vi "Controller Apply BPM Configuration.vi"(8 "Inverse BPM Matrix Mapping":u32[][](array[numeric]), 9 "BPM Configuration Status Out":refnum<notifier>, 10 "BPM Configuration Status In":refnum<notifier>, 11 "Acquisition Network In":T1) -> (2 "Changed?":bool, 3 "Acquisition Network Out":T1)   [LabVIEW 2011, in "Controller VIs.lvlib"]
uses:
  Controller VIs.lvlib
  Types Definitions/Type Acquisition Network Configuration.ctl
  Type Definitions.lvlib
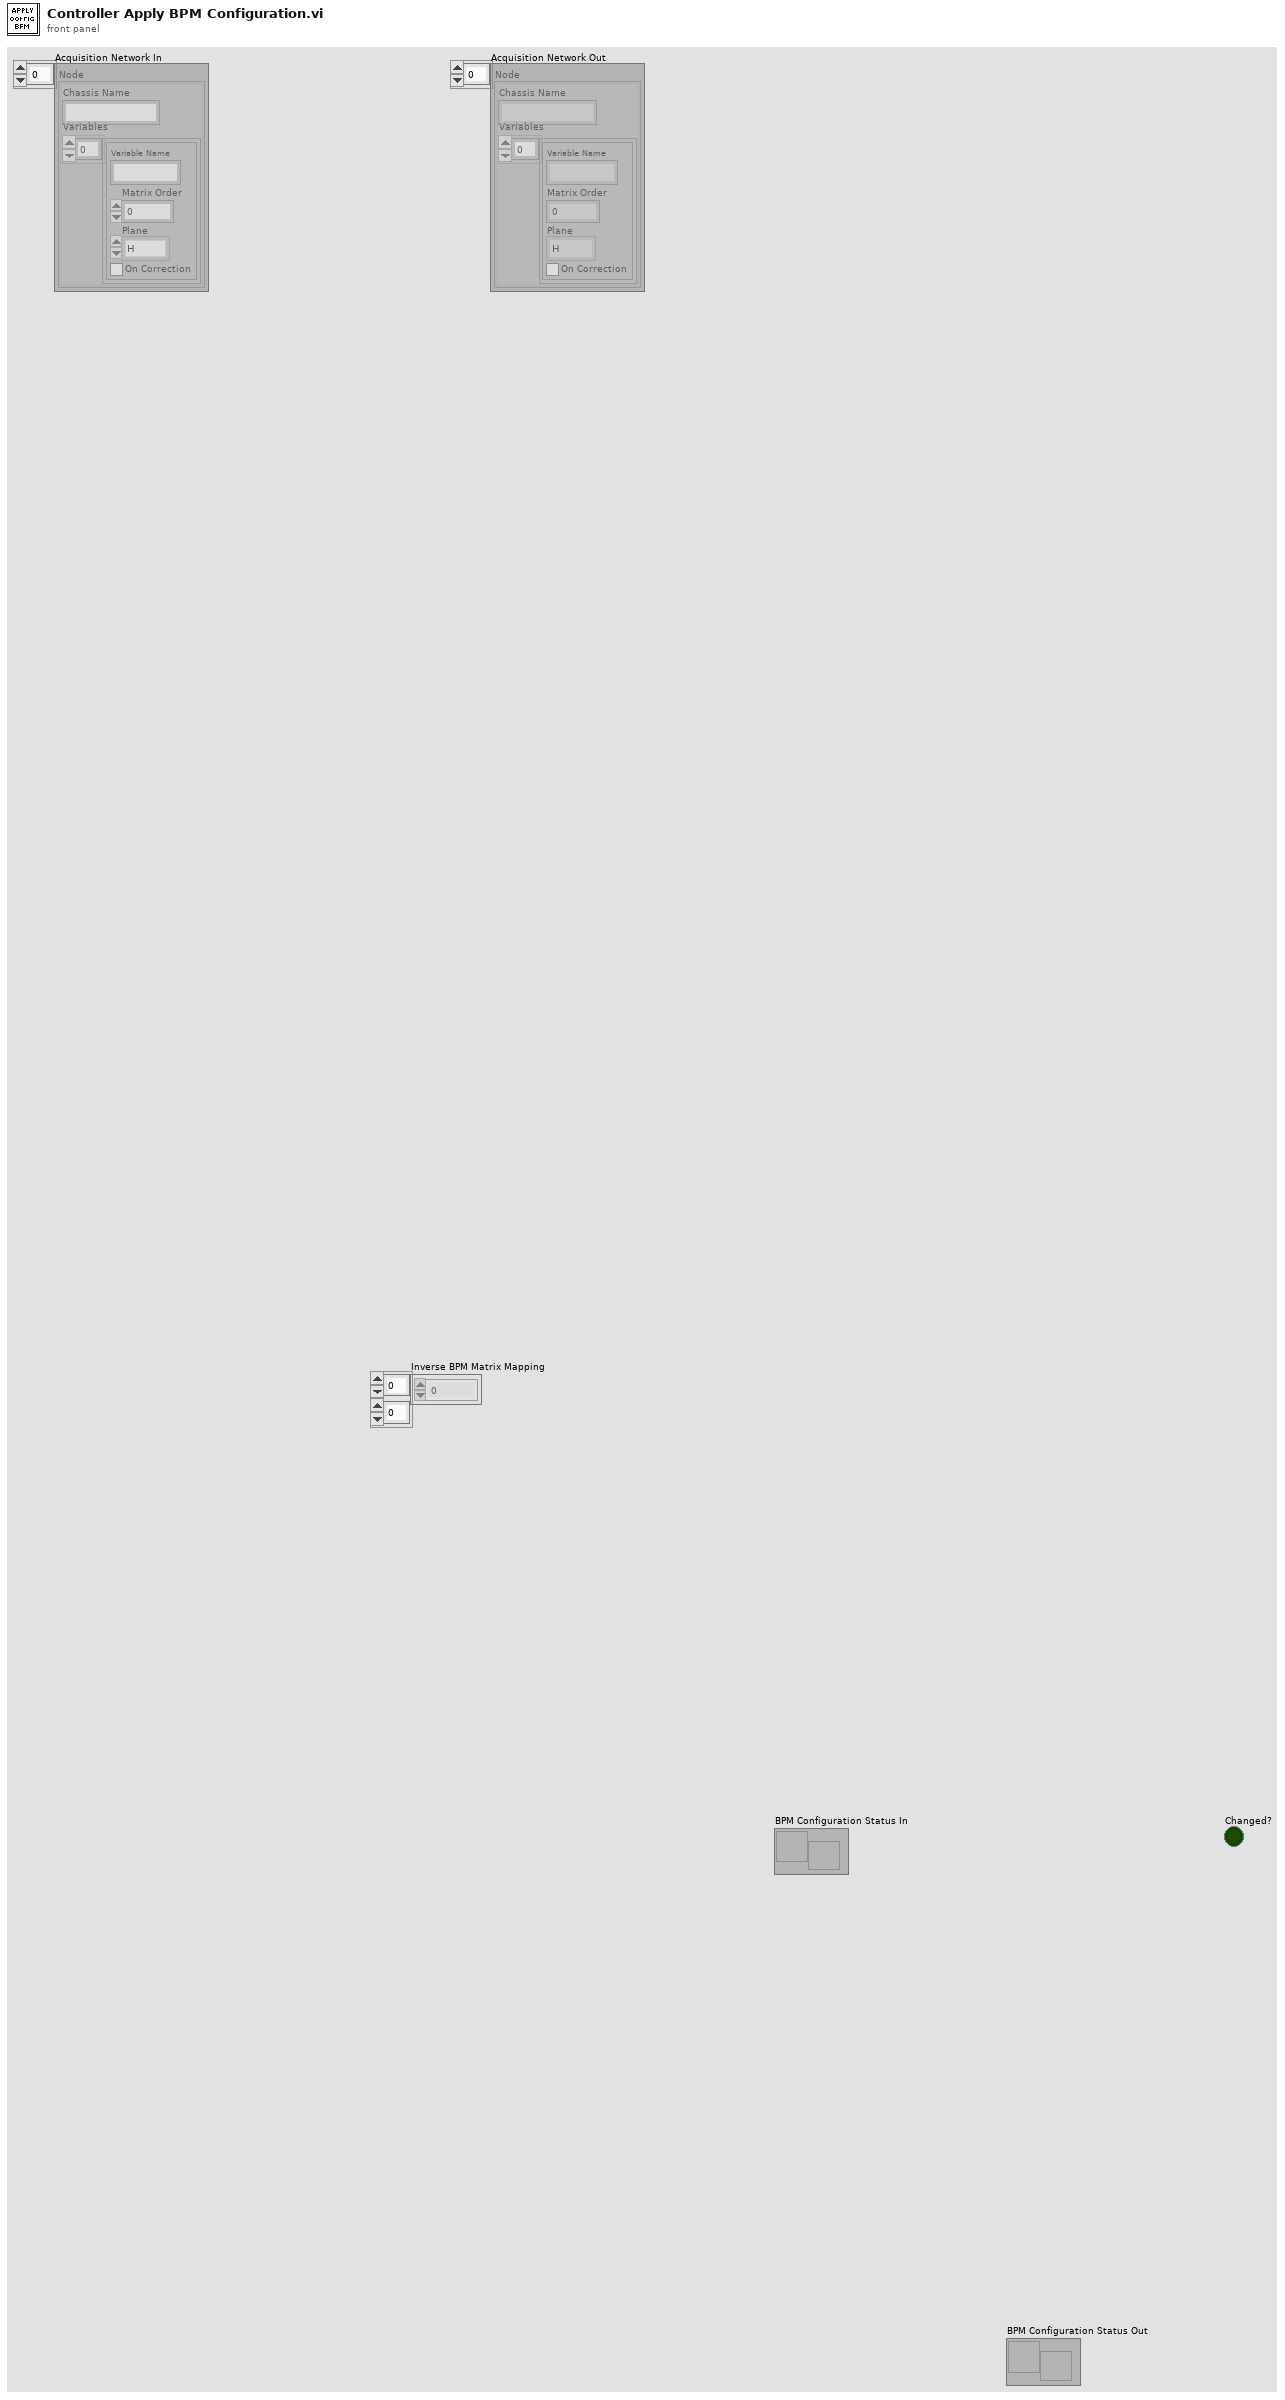
[diagram p1: front panel]
types:
  T1 = typedef "Type Definitions.lvlib/Type Acquisition Network Configuration.ctl" = cluster{"Chassis Name":string, "Variables":cluster{"Variable Name":string, "Matrix Order":u32, "Plane":enum8{"H", "V"}, "On Correction":bool}[]}[]
  T2 = cluster{"Chassis Name":string, "Variables":cluster{"Variable Name":string, "Matrix Order":u32, "Plane":enum8{"H", "V"}, "On Correction":bool}[]}
  T3 = cluster{"Variable Name":string, "Matrix Order":u32, "Plane":enum8{"H", "V"}, "On Correction":bool}[]
  T4 = cluster{"Variable Name":string, "Matrix Order":u32, "Plane":enum8{"H", "V"}, "On Correction":bool}
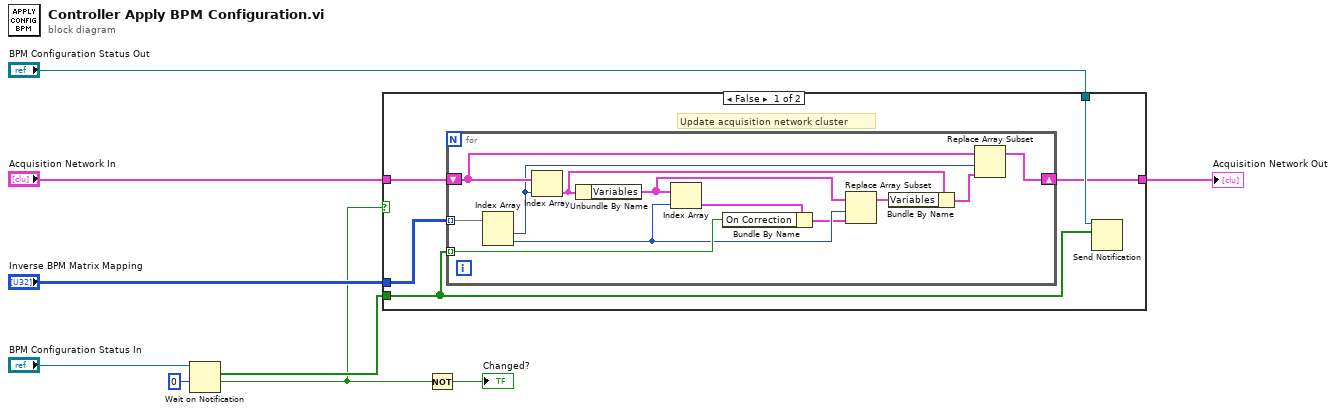
[diagram p0: block diagram]
diagram:
  n1 = Wait on Notification(notifier="BPM Configuration Status In", timeout in ms (-1)=0) -> (notification=w5:bool[], timed out?=w1:bool)  [unwired: 2 in, 2 out]
  n2 = case shown="False" w1 {
    tunnel: "Acquisition Network In" -> [w13 w27]
    tunnel: [w12 w27] -> w3
    tunnel: "BPM Configuration Status Out" -> [w14 _]
    tunnel: w5 -> [w10 _]
    tunnel: "Inverse BPM Matrix Mapping" -> [w11 _]
    frame False {
      # "Update acquisition network cluster"
      n3 = for {
        tunnel: w11 -> [w26] mode=indexing
        tunnel: w10 -> [w24] mode=indexing
        shift-right: [w15] -> w12
        shift-left: w13 -> [w23]
        n4 = Index Array(array=w26) -> (element #1=w22:u32, element #2=w20:u32)  [unwired: 2 in]
        n5 = Index Array(array=w23, index=w22) -> (element=w18:T2)
        n6 = Unbundle By Name(w18) -> ("Variables"=w21:T3)
        n7 = Index Array(array=w21, index=w20) -> (element=w25:T4)
        n8 = Bundle By Name(cluster=w25, "On Correction"=w24) -> (w19:T4)
        n9 = Replace Array Subset(array=w21, new element=w19, index=w20) -> (w17:T3)
        n10 = Bundle By Name(cluster=w18, "Variables"=w17) -> (w16:T2)
        n11 = Replace Array Subset(array=w23, new element=w16, index=w22) -> (w15:T1)
      }
      n12 = Send Notification(notification=w10, notifier=w14) -> ()  [unwired: 1 in, 2 out]
    }
    frame True {
    }
  }
  "Acquisition Network Out" <- w3
  n13 = Not(x=w1) -> (.not. x?=→"Changed?":bool)
